vi "ConfigDevice.vi"(8 "error in (no error)":errorcluster, 11 "NhRegenGridSim in":refnum<class "NHRGridSim.lvclass">) -> (0 "error out":errorcluster, 3 "NhRegenGridSim out":refnum<class "NHRGridSim.lvclass">)   [LabVIEW 2018, in "AcPwrPlugins.lvlib" / "NHRGridSim.lvclass"]
doc: "This VI configures the instrument for the properties set such as instrument mode, slew, power level, etc."
uses:
  NHRGridSim.lvclass
  TypeDefs/ConfigDevicesTypeDef.ctl
  TypeDefs/RangeCheck.ctl
  <vilib>/Utility/error.llb/Error Cluster From Error Code.vi
  <instrlib>/NH Research 9400 Series/Public/Configure/Configure Range (Voltage).vi
  <instrlib>/NH Research 9400 Series/Public/Configure/Configure Range (Current).vi
  <instrlib>/NH Research 9400 Series/Public/Configure/Configure Slew Rate (Multi Phase).vi
  <instrlib>/NH Research 9400 Series/Public/Configure/Configure Slew Rate (Frequency).vi
  <instrlib>/NH Research 9400 Series/Public/Configure/Configure Slew Rate (Power).vi
  <instrlib>/NH Research 9400 Series/Public/Configure/Configure Slew Rate (Voltage).vi
  <instrlib>/NH Research 9400 Series/Public/Configure/Configure Slew Rate (Current).vi
  <instrlib>/NH Research 9400 Series/Public/Configure/Configure Setpoint (Power).vi
  <instrlib>/NH Research 9400 Series/Public/Configure/Configure Setpoint (Current).vi
  <instrlib>/NH Research 9400 Series/Public/Configure/Configure Setpoint (Voltage).vi
  <instrlib>/NH Research 9400 Series/Public/Configure/Configure Setpoint (Frequency).vi
  <vilib>/ErrorRing/Error Ring.xnode
  <instrlib>/NH Research 9400 Series/NH Research 9400 Series.lvlib
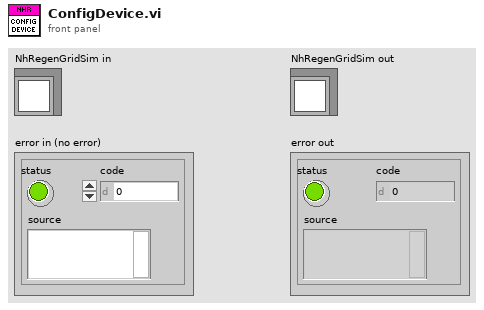
[diagram p1: front panel]
types:
  T1 = typedef "AcPwrPlugins.lvlib/NHRGridSim.lvclass/ConfigDevicesTypeDef.ctl" = enum16{"Error", "SelectMode", "PhaseName", "Safety", "Range", "Slew", "SetPoints", "Measurement"}
  T2 = typedef "AcPwrPlugins.lvlib/NHRGridSim.lvclass/DeviceSettings.ctl" = cluster{"SlewRates":cluster{"Islew":dbl, "Vslew":dbl, "Pslew":dbl, "FreqSlew":dbl, "AngleABSlew":dbl, "AngleACSlew":dbl}, "Phases":cluster{"Pout (W)":dbl, "Iout (A)":dbl, "PhaseAngle":dbl, "Vout (V)":dbl, "Phase Name":string}[], "Measurement":cluster{"ApertureLength (s)":dbl, "NumberOfSamples":u32}, "Ranges":cluster{"Irange (A)":dbl, "Vrange (V)":dbl}, "Mode":enum8{"One 3-Phase AC", "One AC", "One DC", "Three AC", "Three DC", "One 2-Phase AC and One AC", "One 2-Phase AC and One DC", "Two AC", "One AC and One DC", "Two AC and One DC", "One AC and Two DC", "One DC and One AC", "Two DC"}, "PowerMax":u16, "TransformerRatio":dbl, "Waveshape":dbl[], "Handle":string, "FreqOut (Hz)":dbl, "Connected":bool, "Safety Limits":cluster{"Minimum Voltage (V)":dbl, "Minimum Voltage Time (s)":dbl, "Maximum Voltage (V)":dbl, "Maximum Voltage Time (s)":dbl, "Maximum Source Amps (A)":dbl, "Maximum Source Amps Time (s)":dbl, "Maximum Sink Amps (A)":dbl, "Maximum Sink Amps Time (s)":dbl, "Maximum Source Power (W)":dbl, "Maximum Source Power Time (s)":dbl, "Maximum Sink Power (W)":dbl, "Maximum Sink Power Time (s)":dbl, "Peak Voltage (V)":dbl, "Peak Voltage Enable":bool, "Peak Amps (A)":dbl, "Peak Amps Enable":bool}, "btnIdQuery":bool, "btnReset":bool, "Initialize Timeout (10000 ms)":u32}[]
  T3 = enum8{"One 3-Phase AC", "One AC", "One DC", "Three AC", "Three DC", "One 2-Phase AC and One AC", "One 2-Phase AC and One DC", "Two AC", "One AC and One DC", "Two AC and One DC", "One AC and Two DC", "One DC and One AC", "Two DC"}
  T4 = cluster{"Pout (W)":dbl, "Iout (A)":dbl, "PhaseAngle":dbl, "Vout (V)":dbl, "Phase Name":string}[]
  T5 = cluster{"Minimum Voltage (V)":dbl, "Minimum Voltage Time (s)":dbl, "Maximum Voltage (V)":dbl, "Maximum Voltage Time (s)":dbl, "Maximum Source Amps (A)":dbl, "Maximum Source Amps Time (s)":dbl, "Maximum Sink Amps (A)":dbl, "Maximum Sink Amps Time (s)":dbl, "Maximum Source Power (W)":dbl, "Maximum Source Power Time (s)":dbl, "Maximum Sink Power (W)":dbl, "Maximum Sink Power Time (s)":dbl, "Peak Voltage (V)":dbl, "Peak Voltage Enable":bool, "Peak Amps (A)":dbl, "Peak Amps Enable":bool}
  T6 = typedef "AcPwrPlugins.lvlib/NHRGridSim.lvclass/RangeCheck.ctl" = enum16{"SlewCurrent", "SlewVoltage", "SlewPower", "SlewFrequency", "ApertureLength", "NumberOfSamples", "SlewAngleMultiPhaseAB", "SlewAngleMultiPhaseAC", "VoltageRange", "CurrentRange", "PhaseAngle", "Power", "Current", "Voltage", "Frequency"}[]
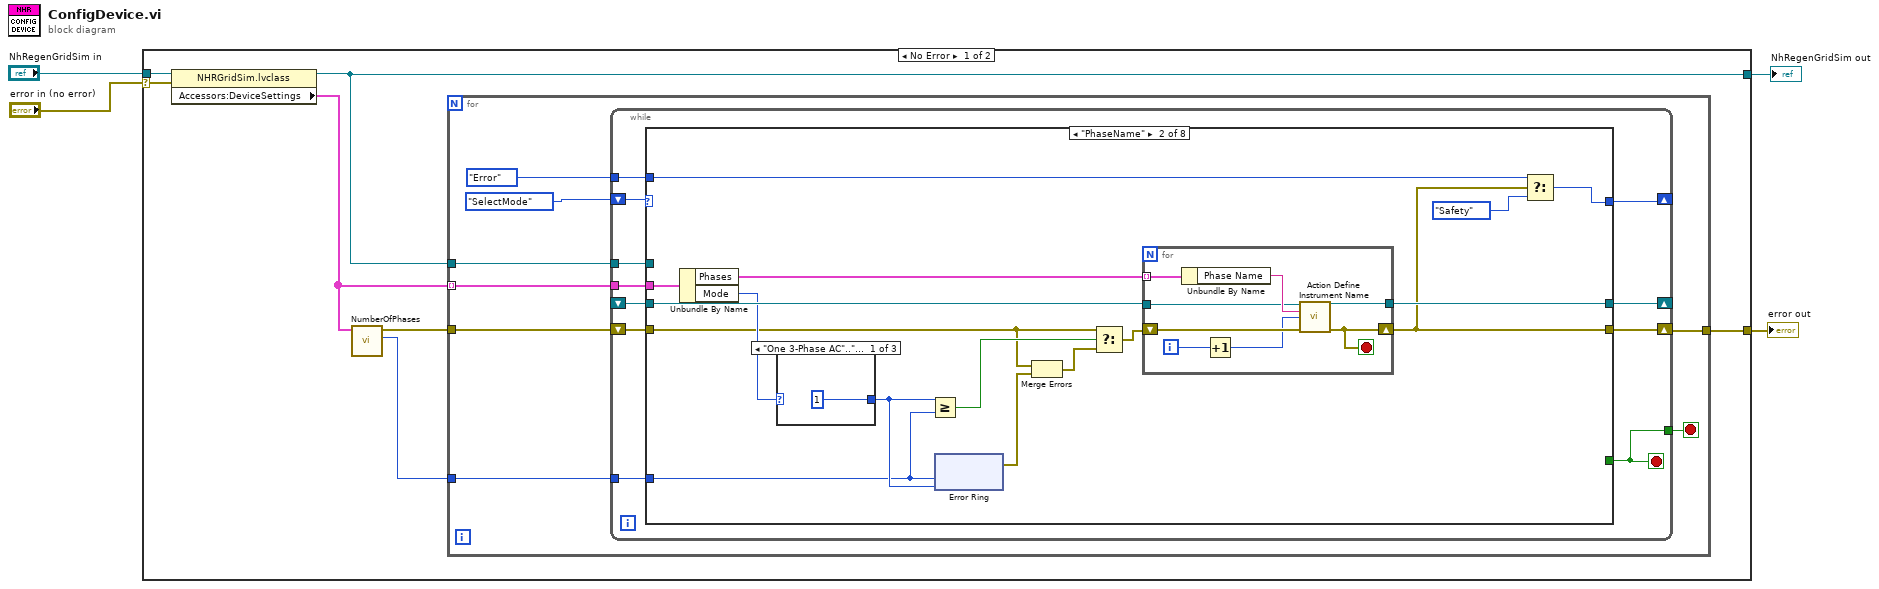
[diagram p0: block diagram]
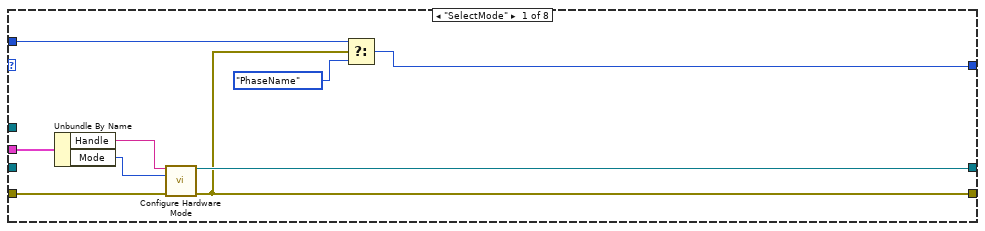
[diagram p2: hidden frame]
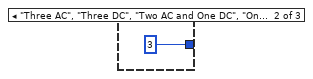
[diagram p3: hidden frame]
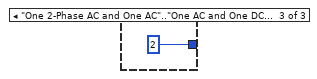
[diagram p4: hidden frame]
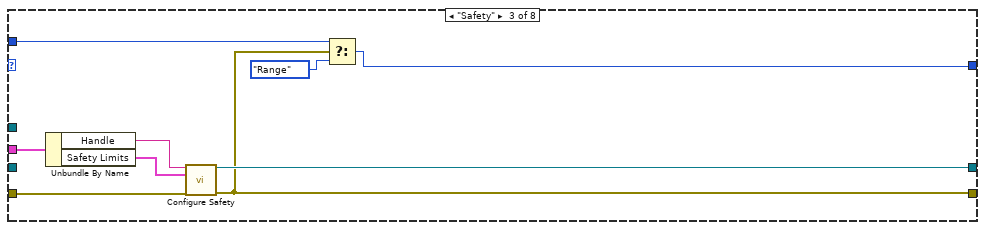
[diagram p5: hidden frame]
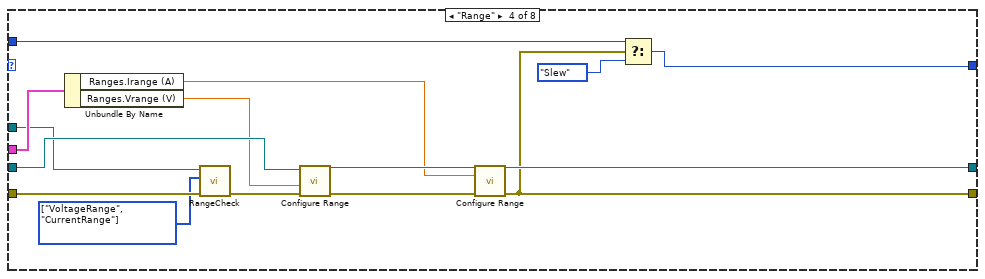
[diagram p6: hidden frame]
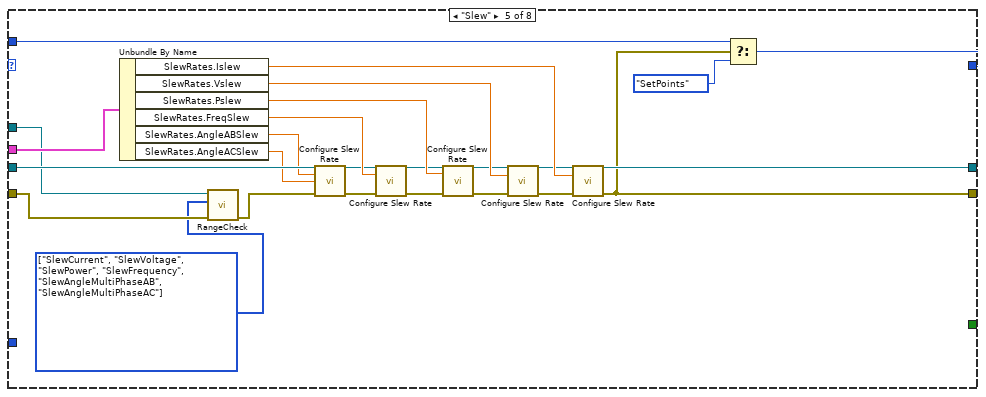
[diagram p7: hidden frame]
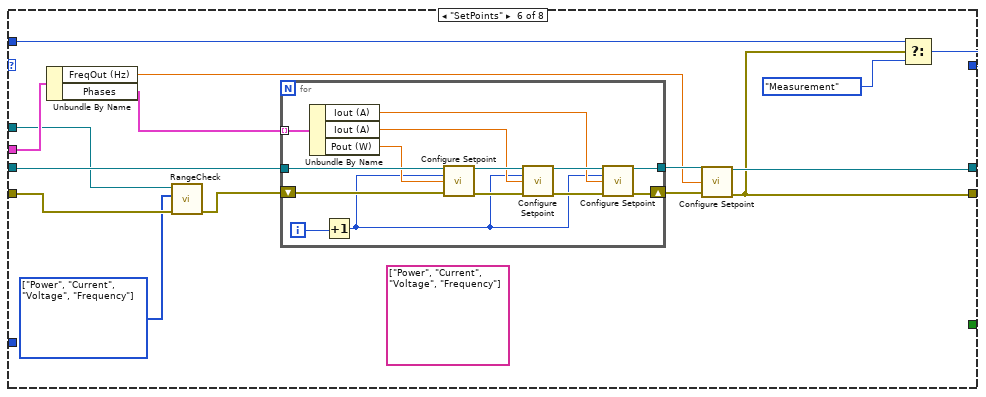
[diagram p8: hidden frame]
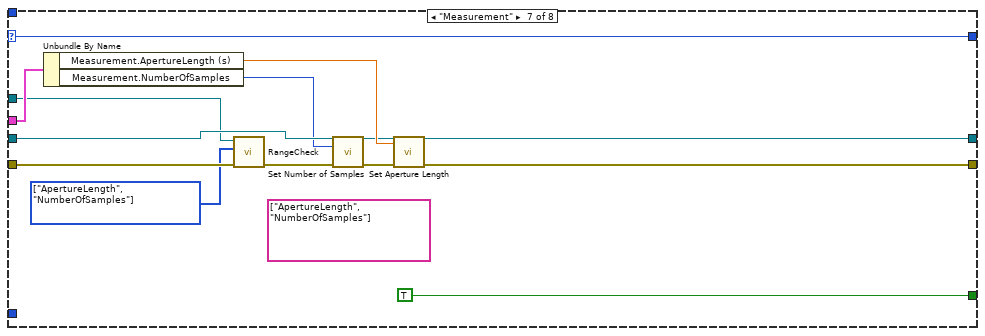
[diagram p9: hidden frame]
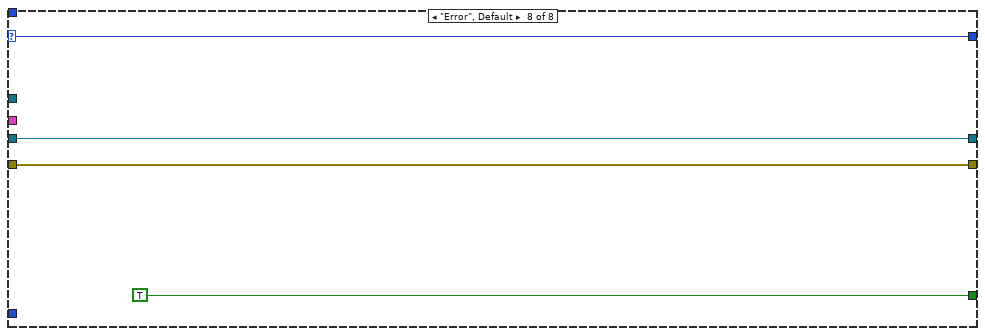
[diagram p10: hidden frame]
diagram:
  n1 = case shown="No Error" "error in (no error)" {
    selector: "error in (no error)" -> [w10 w171]
    tunnel: "NhRegenGridSim in" -> [w11 w172]
    tunnel: [w9 w172] -> w2
    tunnel: [w8 w171] -> w1
    frame No Error {
      n2 = property class="NHRGridSim.lvclass"(reference=w11, error in=w10) -> (reference out=w9:refnum<class "NHRGridSim.lvclass">, "Accessors:DeviceSettings"=w7:T2)  [unwired: 1 out]
      n3 = call "NumberOfPhases.vi"("DeviceSettings"=w7) -> ("NumberOfPhases"=w5:i32, "error out"=w6:errorcluster)  [unwired: 8 in, 1 out]
      n4 = for {
        tunnel: w7 -> [w15] mode=indexing
        tunnel: w9 -> [w19]
        tunnel: w6 -> [w18]
        tunnel: [w17] -> w8
        tunnel: w5 -> [w12]
        stop <- w16 stop-if-true
        n5 = while {
          shift-right: [w28] -> _
          shift-left: ConfigDevicesTypeDef."SelectMode" ("AcPwrPlugins.lvlib:NhRegenGridSim.lvclass:ConfigDevicesTypeDef") -> [w22]
          tunnel: w15 -> [w29]
          tunnel: w19 -> [w30]
          shift-right: [w26] -> w17
          shift-left: w18 -> [w27]
          shift-right: [w25] -> _
          shift-left: _ -> [w24]
          tunnel: [w23] -> w16
          tunnel: ConfigDevicesTypeDef."Error" ("AcPwrPlugins.lvlib:NhRegenGridSim.lvclass:ConfigDevicesTypeDef") -> [w21]
          tunnel: w12 -> [w20]
          stop <- w23 stop-if-true
          n6 = case shown="\"PhaseName\"" w22 {
            selector: w22 -> [_ _ _ _ _ _ w155 w169]
            tunnel: w30 -> [_ _ _ w89 w104 w129 w159 _]
            tunnel: w29 -> [w39 w55 w83 w96 w107 w137 w165 _]
            tunnel: [w38 w43 w78 w88 w103 w128 w155 w169] -> w28
            tunnel: w27 -> [w37 w45 w81 w91 w106 w131 w157 w168]
            tunnel: [w33 w44 w75 w86 w101 w126 w156 w168] -> w26
            tunnel: [w35 w54 w80 w94 w123 w135 w162 w167] -> w25
            tunnel: w24 -> [_ w52 _ w95 w122 w138 w161 w167]
            tunnel: [_ _ _ _ _ _ TRUE TRUE] -> w23
            tunnel: w21 -> [w32 w41 w77 w87 w102 w127 _ _]
            tunnel: w20 -> [_ w40 _ _ _ _ _ _]
            frame "SelectMode" {
              n7 = Unbundle By Name(w39) -> ("Handle"=w36:string, "Mode"=w34:T3)
              n8 = call <instrlib>:"Configure Hardware Mode.vi"("VISA resource name"=w36, "Mode"=w34, "error in (no error)"=w37) -> ("VISA resource name out"=w35:refnum<visa-resource-name>, "error out"=w33:errorcluster)  [unwired: 11 in]
              n9 = Select(t=w32, s=w33, f=ConfigDevicesTypeDef."PhaseName" ("AcPwrPlugins.lvlib:NhRegenGridSim.lvclass:ConfigDevicesTypeDef")) -> (s? t:f=w38:T1)
            }
            frame "PhaseName" {
              n10 = Unbundle By Name(w55) -> ("Phases"=w53:T4, "Mode"=w51:T3)
              n11 = case shown="\"One 3-Phase AC\"..\"One DC\", Default" w51 {
                tunnel: [1 3 2] -> w47
                frame "One 3-Phase AC".."One DC", Default {
                }
                frame "Three AC", "Three DC", "Two AC and One DC", "One AC and Two DC" {
                }
                frame "One 2-Phase AC and One AC".."One AC and One DC", "One DC and One AC", "Two DC" {
                }
              }
              n12 = Greater Or Equal?(x=w47, y=w40) -> (x >= y?=w50:bool)
              n13 = xnode "Error Ring"("parameter 0"=w40, "parameter 1"=w47) -> ("error out"=w46:errorcluster)
              n14 = Merge Errors(w45, w46) -> (w48:errorcluster)
              n15 = Select(t=w45, s=w50, f=w48) -> (s? t:f=w49:errorcluster)
              n16 = for {
                tunnel: [w73] -> w54
                shift-right: [w69] -> w44
                shift-left: w49 -> [w74]
                tunnel: w52 -> [w70]
                tunnel: w53 -> [w72] mode=indexing
                i -> [w68]
                stop <- w69 stop-if-true
                n17 = Unbundle By Name(w72) -> ("Phase Name"=w71:string)
                n18 = Increment(x=w68) -> (x+1=w67:i32)
                n19 = call <instrlib>:"Action Define Instrument Name.vi"("VISA resource name"=w70, "Logical Instrument Name"=w71, "Logical Instrument Number"=w67, "error in (no error)"=w74) -> ("VISA resource name out"=w73:refnum<visa-resource-name>, "error out"=w69:errorcluster)  [unwired: 10 in]
              }
              n20 = Select(t=w41, s=w44, f=ConfigDevicesTypeDef."Safety" ("AcPwrPlugins.lvlib:NhRegenGridSim.lvclass:ConfigDevicesTypeDef")) -> (s? t:f=w43:T1)
            }
            frame "Safety" {
              n21 = Unbundle By Name(w83) -> ("Handle"=w82:string, "Safety Limits"=w79:T5)
              n22 = call <instrlib>:"Configure Safety.vi"("VISA resource name"=w82, "Safety Limits"=w79, "error in (no error)"=w81) -> ("VISA resource name out"=w80:refnum<visa-resource-name>, "error out"=w75:errorcluster)  [unwired: 11 in]
              n23 = Select(t=w77, s=w75, f=ConfigDevicesTypeDef."Range" ("AcPwrPlugins.lvlib:NhRegenGridSim.lvclass:ConfigDevicesTypeDef")) -> (s? t:f=w78:T1)
            }
            frame "Range" {
              w84 = T6 [enum."VoltageRange", enum."CurrentRange"] items=["SlewCurrent", "SlewVoltage", "SlewPower", "SlewFrequency", "ApertureLength", "NumberOfSamples", "SlewAngleMultiPhaseAB", "SlewAngleMultiPhaseAC", "VoltageRange", "CurrentRange", "PhaseAngle", "Power", "Current", "Voltage", "Frequency"] ("RangeCheck")
              n24 = Unbundle By Name(w96) -> ("Ranges.Irange (A)"=w92:dbl, "Ranges.Vrange (V)"=w93:dbl)
              n25 = call-dynamic "RangeCheck.vi"("NhRegenGridSim in"=w89, "RangeCheck"=w84, "error in (no error)"=w91) -> ("error out"=w90:errorcluster)  [unwired: 6 in, 1 out]
              n26 = call-poly <instrlib>:"Configure Range.vi"("VISA resource name"=w95, "Voltage Range (0 V)"=w93, "error in (no error)"=w90) -> ("VISA resource name out"=w97:refnum<visa-resource-name>, "error out"=w98:errorcluster)  [unwired: 11 in]
              n27 = call-poly <instrlib>:"Configure Range.vi"("VISA resource name"=w97, "Current Range (0 A)"=w92, "error in (no error)"=w98) -> ("VISA resource name out"=w94:refnum<visa-resource-name>, "error out"=w86:errorcluster)  [unwired: 11 in]
              n28 = Select(t=w87, s=w86, f=ConfigDevicesTypeDef."Slew" ("AcPwrPlugins.lvlib:NhRegenGridSim.lvclass:ConfigDevicesTypeDef")) -> (s? t:f=w88:T1)
            }
            frame "Slew" {
              w99 = T6 [enum."SlewCurrent", enum."SlewVoltage", enum."SlewPower", enum."SlewFrequency", enum."SlewAngleMultiPhaseAB", enum."SlewAngleMultiPhaseAC"] items=["SlewCurrent", "SlewVoltage", "SlewPower", "SlewFrequency", "ApertureLength", "NumberOfSamples", "SlewAngleMultiPhaseAB", "SlewAngleMultiPhaseAC", "VoltageRange", "CurrentRange", "PhaseAngle", "Power", "Current", "Voltage", "Frequency"] ("RangeCheck")
              n29 = Unbundle By Name(w107) -> ("SlewRates.Islew"=w120:dbl, "SlewRates.Vslew"=w119:dbl, "SlewRates.Pslew"=w117:dbl, "SlewRates.FreqSlew"=w115:dbl, "SlewRates.AngleABSlew"=w114:dbl, "SlewRates.AngleACSlew"=w113:dbl)
              n30 = call-dynamic "RangeCheck.vi"("NhRegenGridSim in"=w104, "RangeCheck"=w99, "error in (no error)"=w106) -> ("error out"=w105:errorcluster)  [unwired: 6 in, 1 out]
              n31 = call-poly <instrlib>:"Configure Slew Rate.vi"("VISA resource name"=w122, "Slew Rate Phase Angle A to B (0 degrees per sec)"=w114, "Slew Rate Phase Angle A to C (0 degrees per sec)"=w113, "error in (no error)"=w105) -> ("VISA resource name out"=w111:refnum<visa-resource-name>, "error out"=w112:errorcluster)  [unwired: 10 in]
              n32 = call-poly <instrlib>:"Configure Slew Rate.vi"("VISA resource name"=w111, "Frequency Slew (0 Hz per sec)"=w115, "error in (no error)"=w112) -> ("VISA resource name out"=w110:refnum<visa-resource-name>, "error out"=w116:errorcluster)  [unwired: 11 in]
              n33 = call-poly <instrlib>:"Configure Slew Rate.vi"("VISA resource name"=w110, "Power Slew Rate (0 W per sec)"=w117, "error in (no error)"=w116) -> ("VISA resource name out"=w109:refnum<visa-resource-name>, "error out"=w118:errorcluster)  [unwired: 11 in]
              n34 = call-poly <instrlib>:"Configure Slew Rate.vi"("VISA resource name"=w109, "Voltage Slew Rate (0 V per sec)"=w119, "error in (no error)"=w118) -> ("VISA resource name out"=w108:refnum<visa-resource-name>, "error out"=w121:errorcluster)  [unwired: 11 in]
              n35 = call-poly <instrlib>:"Configure Slew Rate.vi"("VISA resource name"=w108, "Current Slew Rate (0 A per sec)"=w120, "error in (no error)"=w121) -> ("VISA resource name out"=w123:refnum<visa-resource-name>, "error out"=w101:errorcluster)  [unwired: 11 in]
              n36 = Select(t=w102, s=w101, f=ConfigDevicesTypeDef."SetPoints" ("AcPwrPlugins.lvlib:NhRegenGridSim.lvclass:ConfigDevicesTypeDef")) -> (s? t:f=w103:T1)
            }
            frame "SetPoints" {
              w124 = T6 [enum."Power", enum."Current", enum."Voltage", enum."Frequency"] items=["SlewCurrent", "SlewVoltage", "SlewPower", "SlewFrequency", "ApertureLength", "NumberOfSamples", "SlewAngleMultiPhaseAB", "SlewAngleMultiPhaseAC", "VoltageRange", "CurrentRange", "PhaseAngle", "Power", "Current", "Voltage", "Frequency"] ("RangeCheck")
              (unwired) string[] ["Power", "Current", "Voltage", "Frequency"]
              n37 = Unbundle By Name(w137) -> ("FreqOut (Hz)"=w132:dbl, "Phases"=w136:T4)
              n38 = call-dynamic "RangeCheck.vi"("NhRegenGridSim in"=w129, "RangeCheck"=w124, "error in (no error)"=w131) -> ("error out"=w130:errorcluster)  [unwired: 6 in, 1 out]
              n39 = for {
                tunnel: w138 -> [w148]
                tunnel: [w140] -> w133
                shift-right: [w139] -> w134
                shift-left: w130 -> [w147]
                tunnel: w136 -> [w146] mode=indexing
                i -> [w142]
                n40 = Unbundle By Name(w146) -> ("Iout (A)"=w143:dbl, "Iout (A)"=w144:dbl, "Pout (W)"=w145:dbl)
                n41 = Increment(x=w142) -> (x+1=w141:i32)
                n42 = call-poly <instrlib>:"Configure Setpoint.vi"("VISA resource name"=w148, "Phase (0: All)"=w141, "Output Power (0 W)"=w145, "error in (no error)"=w147) -> ("VISA resource name out"=w149:refnum<visa-resource-name>, "error out"=w152:errorcluster)  [unwired: 10 in]
                n43 = call-poly <instrlib>:"Configure Setpoint.vi"("VISA resource name"=w149, "Phase (0: All)"=w141, "Output Current (0 A)"=w144, "error in (no error)"=w152) -> ("VISA resource name out"=w150:refnum<visa-resource-name>, "error out"=w151:errorcluster)  [unwired: 10 in]
                n44 = call-poly <instrlib>:"Configure Setpoint.vi"("VISA resource name"=w150, "Phase (0: All)"=w141, "Output Voltage (0 V)"=w143, "error in (no error)"=w151) -> ("VISA resource name out"=w140:refnum<visa-resource-name>, "error out"=w139:errorcluster)  [unwired: 10 in]
              }
              n45 = call-poly <instrlib>:"Configure Setpoint.vi"("VISA resource name"=w133, "Output Frequency (60 Hz)"=w132, "error in (no error)"=w134) -> ("VISA resource name out"=w135:refnum<visa-resource-name>, "error out"=w126:errorcluster)  [unwired: 11 in]
              n46 = Select(t=w127, s=w126, f=ConfigDevicesTypeDef."Measurement" ("AcPwrPlugins.lvlib:NhRegenGridSim.lvclass:ConfigDevicesTypeDef")) -> (s? t:f=w128:T1)
            }
            frame "Measurement" {
              w153 = T6 [enum."ApertureLength", enum."NumberOfSamples"] items=["SlewCurrent", "SlewVoltage", "SlewPower", "SlewFrequency", "ApertureLength", "NumberOfSamples", "SlewAngleMultiPhaseAB", "SlewAngleMultiPhaseAC", "VoltageRange", "CurrentRange", "PhaseAngle", "Power", "Current", "Voltage", "Frequency"] ("RangeCheck")
              (unwired) string[] ["ApertureLength", "NumberOfSamples"]
              n47 = Unbundle By Name(w165) -> ("Measurement.ApertureLength (s)"=w164:dbl, "Measurement.NumberOfSamples"=w160:u32)
              n48 = call-dynamic "RangeCheck.vi"("NhRegenGridSim in"=w159, "RangeCheck"=w153, "error in (no error)"=w157) -> ("error out"=w158:errorcluster)  [unwired: 6 in, 1 out]
              n49 = call <instrlib>:"Set Number of Samples.vi"("VISA resource name"=w161, "Number of Samples"=w160, "error in (no error)"=w158) -> ("VISA resource name out"=w163:refnum<visa-resource-name>, "error out"=w166:errorcluster)  [unwired: 11 in]
              n50 = call <instrlib>:"Set Aperture Length.vi"("VISA resource name"=w163, "Aperture Length (s)"=w164, "error in (no error)"=w166) -> ("VISA resource name out"=w162:refnum<visa-resource-name>, "error out"=w156:errorcluster)  [unwired: 11 in]
            }
            frame "Error", Default {
            }
          }
        }
      }
    }
    frame Error {
    }
  }
  "NhRegenGridSim out" <- w2
  "error out" <- w1
